vi "Config Dev Mode.vi"(8 "error in":errorcluster, 10 "Dev Mode":bool, 11 "VISA resource name":refnum<visa-resource-name>) -> (0 "error out":errorcluster, 3 "VISA resource name out":refnum<visa-resource-name>)   [LabVIEW 2017, in "Andeen-Hagerling 2700.lvlib"]
doc: "Enables or disables the deviation mode. When enabled, the deviation mode takes capacitance and loss measurements very rapidly and converts them to analog voltages that are proportional to the measured capacitance and loss. This is a special mode of operation that functions as a high-speed alternative to the normal bridge mode measurements."
uses:
  Andeen-Hagerling 2700.lvlib
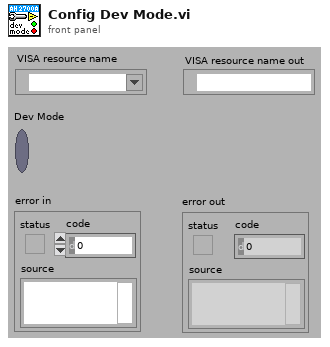
[diagram p1: front panel]
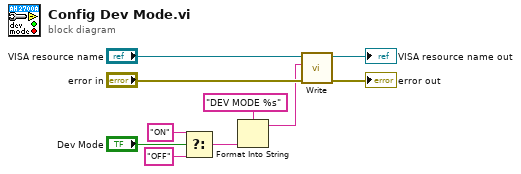
[diagram p0: block diagram]
diagram:
  n1 = Select(t="ON", s="Dev Mode", f="OFF") -> (s? t:f=w1:string)
  n2 = Format Into String(format string="DEV MODE %s", w1) -> (resulting string=w2:string)  [unwired: 2 in, 1 out]
  n3 = call "Write.vi"("error in"="error in", "command"=w2, "VISA resource name"="VISA resource name") -> ("error out"=→"error out":errorcluster, "VISA resource name out"=→"VISA resource name out":refnum<visa-resource-name>)  [unwired: 7 in]
